vi "Launch Actor.vi"(6 "Open Actor Core front panel? (F)":bool, 8 "error in (no error)":errorcluster, 10 "Actor-to-Caller Enqueuer":refnum<class "Message Enqueuer.lvclass">, 11 "Actor":refnum<class "Actor.lvclass">) -> (0 "error out":errorcluster, 3 "Caller-To-Actor Enqueuer":refnum<class "Message Enqueuer.lvclass">)   [LabVIEW 2013, in "Actor Framework.lvlib" / "Actor.lvclass"]
doc: "(<B>Filename</B>: Actor Framework.lvlib:Actor.lvclass:Launch Actor.vi)\n\nLaunches a top-level VI that handles messages for an actor and starts this actor's tasks. This VI returns a reference to the queue you use to send messages to the actor.\n\nThis VI requires the <B>Actor-to-Caller Enqueuer</B> input, which is the reference that allows the launched actor to communicate with the caller. If you are launching the top-level actor, use the Read Enqueuer method to obtain this reference. If you are launching a nested actor, use the Read Self Enqueuer method instead."
uses:
  <vilib>/ActorFramework/Actor/Actor.lvclass
  <vilib>/ActorFramework/Message Enqueuer/Message Enqueuer.lvclass
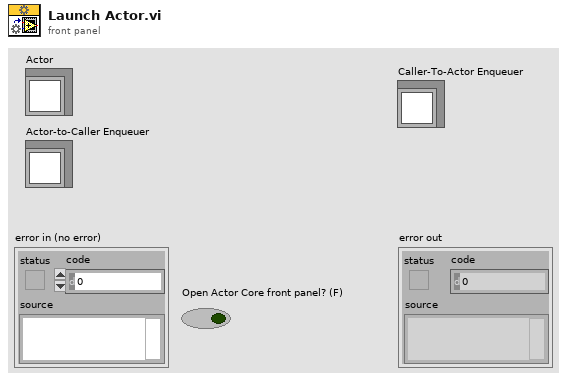
[diagram p1: front panel]
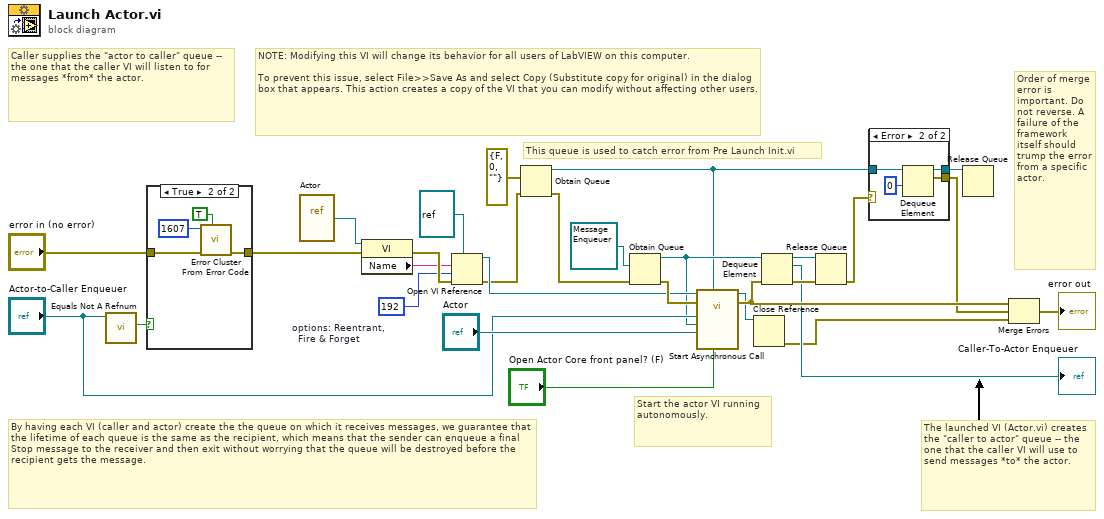
[diagram p0: block diagram]
diagram:
  w20 = 192  # options: Reentrant,       Fire & Forget
  # "This queue is used to catch error from Pre Launch Init.vi"
  # "Order of merge error is important. Do not reverse. A failure of the framework itself should trump the error from a specific actor."
  # "NOTE: Modifying this VI will change its behavior for all users of LabVIEW on this computer.\n\nTo prevent this issue, select File>>Save As and select Copy (Substitute copy for original) in the dialog box that appears. This action creates a copy of the VI that you can modify without affecting other users."
  # "The launched VI (Actor.vi) creates the \"caller to actor\" queue -- the one that the caller VI will use to send messages *to* the actor."
  # "Caller supplies the \"actor to caller\" queue -- the one that the caller VI will listen to for messages *from* the actor."
  # "By having each VI (caller and actor) create the the queue on which it receives messages, we guarantee that the lifetime of each queue is the same as the recipient, which means that the sender can enqueue a final Stop message to the receiver and then exit without worrying that the queue will be destroyed before the recipient gets the message."
  # "Start the actor VI running autonomously."
  n1 = call <vilib>:"Equals Not A Refnum.vi"("Message Enqueuer"="Actor-to-Caller Enqueuer") -> ("Not a refnum?"=w15:bool)  [unwired: 10 in]
  n2 = case shown="True" w15 {
    tunnel: "error in (no error)" -> [w30 w34]
    tunnel: [w30 w33] -> w17
    frame False {
    }
    frame True {
      n3 = call <vilib>:"Error Cluster From Error Code.vi"("show call chain? (False)"=TRUE, "error in (no error)"=w34, "error code (0)"=1607) -> ("error out"=w33:errorcluster)  [unwired: 6 in]
    }
  }
  n4 = vi-ref <vilib>:"Actor.vi"() -> (w23:refnum<vi>)
  n5 = property class="VI"(reference=w23, error in=w17) -> (error out=w22:errorcluster, "Name"=w21:string)  [unwired: 1 out]
  n6 = Open VI Reference(type specifier VI Refnum (for type only)=refnum<vi> refnum, vi path=w21, options=w20, error in (no error)=w22) -> (vi reference=w19:refnum<vi>, error out=w10:errorcluster)  [unwired: 2 in]
  n7 = Obtain Queue(element data type=errorcluster {"status"=FALSE, "code"=0, "source"=""} ("Error"), error in (no error)=w10) -> (queue out=w7:refnum<queue>, error out=w9:errorcluster)  [unwired: 3 in, 1 out]
  n8 = Obtain Queue(element data type=refnum<class "Message Enqueuer.lvclass"> refnum ("Message Enqueuer"), error in (no error)=w9) -> (queue out=w13:refnum<queue>, error out=w28:errorcluster)  [unwired: 3 in, 1 out]
  n9 = call-by-ref "Start Asynchronous Call"(reference=w19, error in=w28, "Open Actor Core front panel? (F)"="Open Actor Core front panel? (F)", "error feedback"=w7, "Actor"="Actor", "queue of queues"=w13, "Send Queue"="Actor-to-Caller Enqueuer") -> (reference out=w3:refnum<vi>, error out=w25:errorcluster)  [unwired: 7 in]
  n10 = Close Reference(reference=w3) -> (error out=w2:errorcluster)  [unwired: 1 in]
  n11 = Dequeue Element(queue=w13, error in (no error)=w25) -> (queue out=w27:refnum<queue>, element=→"Caller-To-Actor Enqueuer":refnum<class "Message Enqueuer.lvclass">, error out=w26:errorcluster)  [unwired: 1 in, 1 out]
  n12 = Release Queue(queue=w27, error in (no error)=w26) -> (error out=w5:errorcluster)  [unwired: 1 in, 2 out]
  n13 = case shown="Error" w5 {
    selector: w5 -> [w36 _]
    tunnel: w7 -> [w35 w40]
    tunnel: [w36 w38] -> w6
    tunnel: [w35 w37] -> w4
    frame No Error {
    }
    frame Error {
      n14 = Dequeue Element(queue=w40, timeout in ms (-1)=0) -> (queue out=w37:refnum<queue>, element=w38:errorcluster)  [unwired: 1 in, 2 out]
    }
  }
  n15 = Release Queue(queue=w4) -> ()  [unwired: 2 in, 3 out]
  n16 = Merge Errors(w25, w6, w2) -> (→"error out":errorcluster)
